vi "mod1 sub.vi"(3 "Modulname":string, 4 "Daten":string, 5 "Format":string="%d") -> (0 "Sperre":bool, 1 "Ausgang":string)   [LabVIEW 2010]
panel:
  out "Zykluslänge b":dbl
  out "Achtung":string
  out "Zykluslänge a":dbl
  out "Pre1A":dbl[][](array[numeric])
  out "TrapA":dbl[][](array[numeric]) format="%.2f"
  out "Main1A":dbl[][](array[numeric]) format="%.2f"
  out "MFC1":dbl[][](array[numeric]) format="%.2f"
  out "FanMain1":dbl[][](array[numeric])
  out "V1B":dbl[][](array[numeric]) format="%.2f"
  out "V1A":dbl[][](array[numeric])
  out "S1A1":dbl[][](array[numeric]) format="%.2f"
  out "pc1 C":dbl[][](array[numeric])
  out "pc1 A":dbl[][](array[numeric])
  in  "TrapA":bool
  in  "FanMain1A":bool
  in  "V1A":bool
  in  "V1B":bool
  in  "Main1A":bool
  in  "Pre1A":bool
  in  "MFC1":bool
  in  "S1A1":bool
  in  "pc1C":bool
  in  "pc1A":bool
  in  "Zurück":bool
  out "new picture":picture
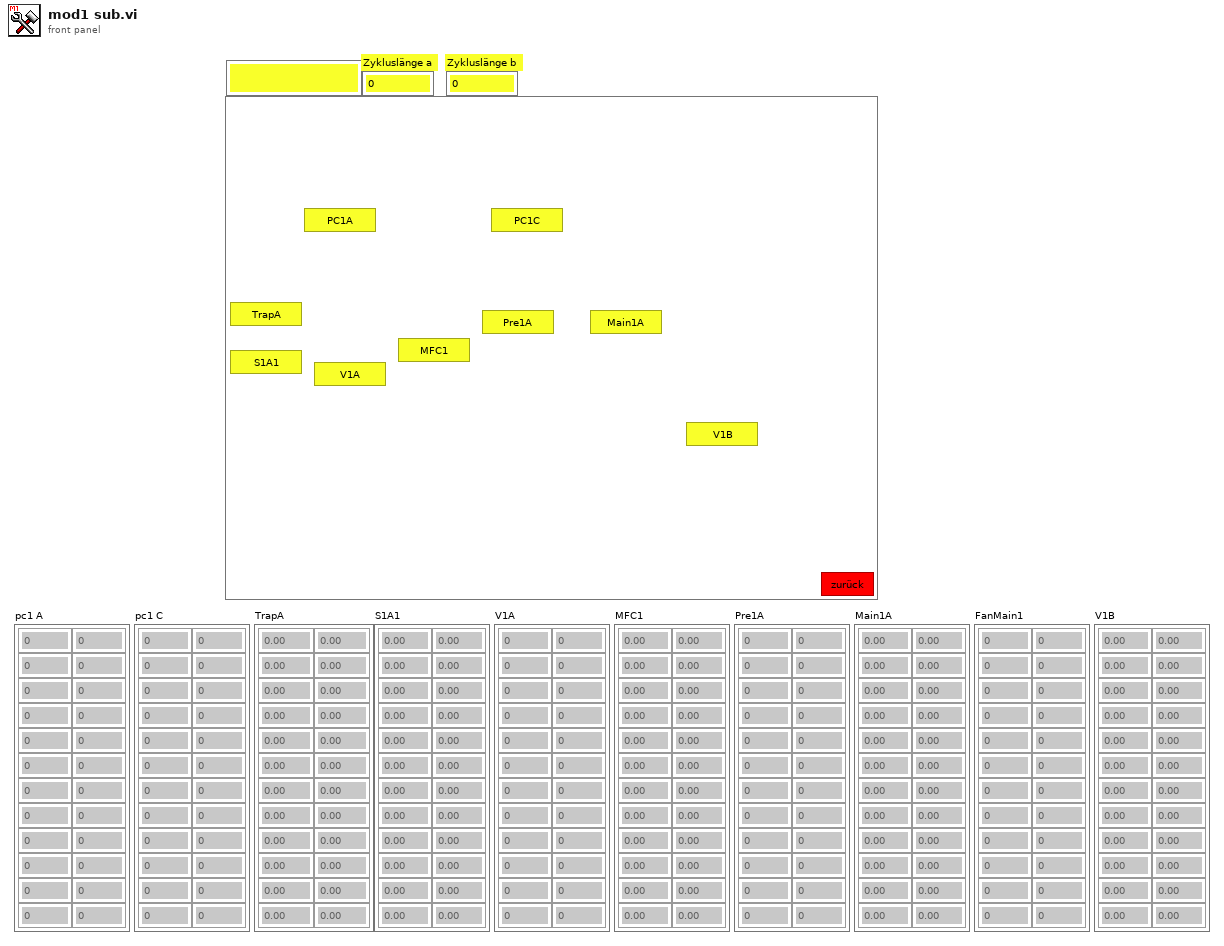
[diagram p1: front panel]
types:
  T1 = typedef "imagedata.ctl" = cluster{"image type":i32, "image depth":i32, "image":u8[], "mask":u8[], "colors":u32[], "Rectangle":cluster{"left":i16, "top":i16, "right":i16, "bottom":i16}}
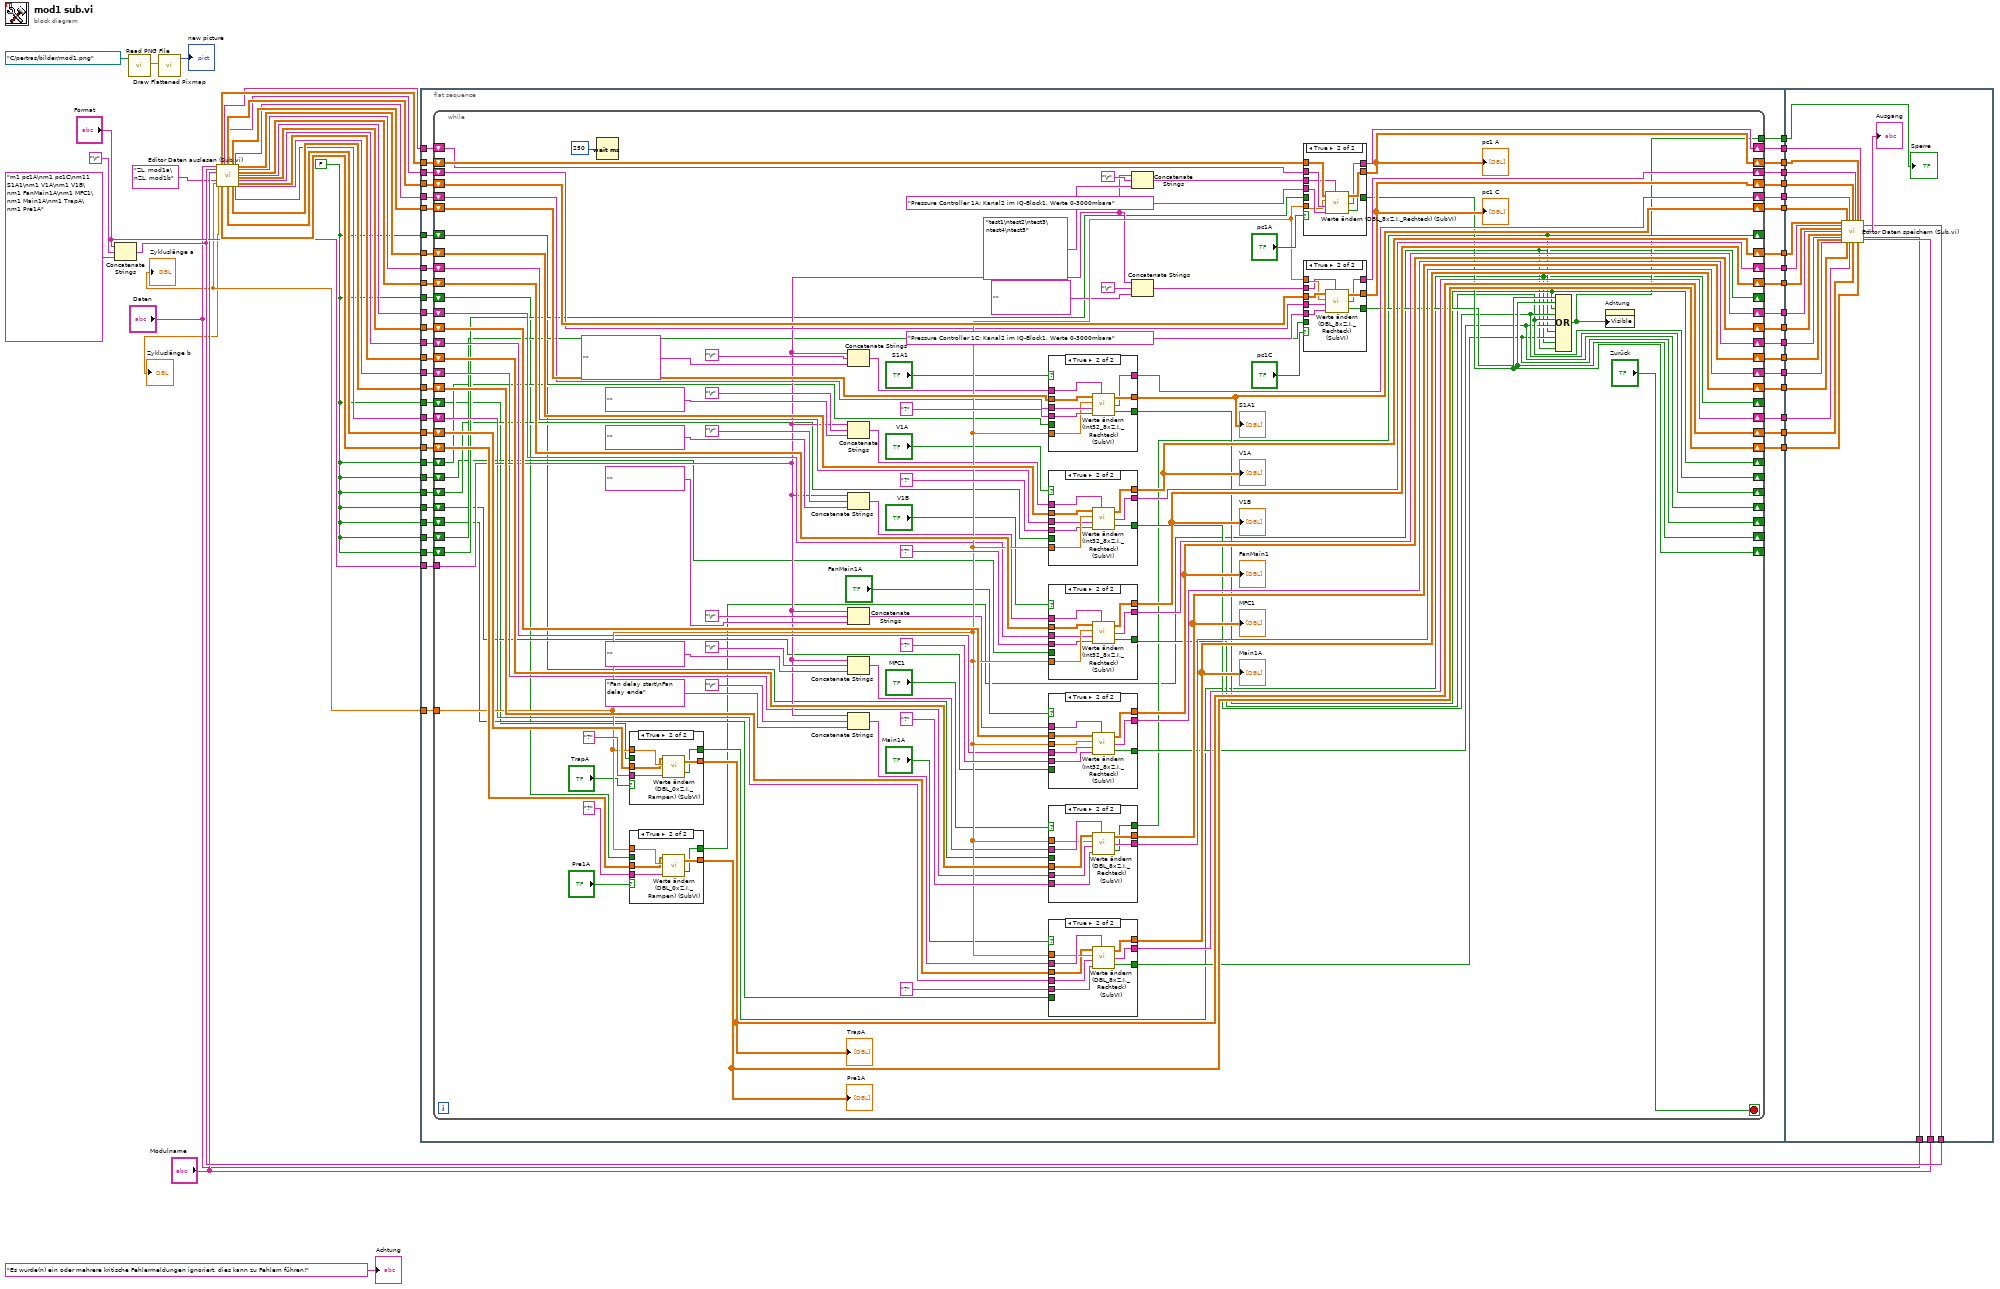
[diagram p0: block diagram]
diagram:
  w2 = FALSE
  n1 = Concatenate Strings("Format", "\r", "m1 pc1A\nm1 pc1C\nm11 S1A1\nm1 V1A\nm1 V1B\nm1 FanMain1A\nm1 MFC1\nm1 Main1A\nm1 TrapA\nm1 Pre1A" ("String")) -> (w38:string)
  n2 = call <vilib>:"Read PNG File.vi"("path to PNG file"=path "C:/pertras/bilder/mod1.png") -> ("image data"=w49:T1)  [unwired: 8 in, 2 out]
  n3 = call <vilib>:"Draw Flattened Pixmap.vi"("image data"=w49) -> ("new picture"=→"new picture":picture)  [unwired: 8 in]
  n4 = call "Editor Daten auslesen (Sub.vi).vi"("Daten"="Daten", "Formatierung+Namen"=w38, "Modulname"="Modulname", "Zykluslängen Namen"="ZL. mod1a\nZL. mod1b" ("Zykluslänge Name")) -> ("Zykluslänge 1"=w10:dbl, "Zykluslänge 2"=→"Zykluslänge b":dbl, "1"=w35:dbl[][], "10"=w21:dbl[][], "Z 1"=w34:string, "2"=w33:dbl[][], "9"=w22:dbl[][], "Z 2"=w32:string, "3"=w31:dbl[][], "8"=w23:dbl[][], "Z 3"=w30:string, "Z 8"=w5:string, "4"=w29:dbl[][], "Z 4"=w20:string, "5"=w28:dbl[][], "Z5"=w27:string, "6"=w26:dbl[][], "Z 6"=w25:string, "7"=w24:dbl[][], "Z 7"=w6:string)  [unwired: 2 in, 2 out]
  "Zykluslänge a" <- w10
  n5 = flat-sequence {
    tunnel: w10 -> [w100]
    tunnel: [w99] -> w48
    tunnel: [w98] -> w47
    tunnel: [w97] -> w46
    tunnel: [w96] -> w45
    tunnel: [w95] -> w44
    tunnel: [w94] -> w43
    tunnel: [w93] -> w42
    tunnel: [w92] -> w41
    tunnel: [w91] -> w40
    tunnel: [w90] -> w39
    tunnel: w35 -> [w89]
    tunnel: w34 -> [w88]
    tunnel: w33 -> [w87]
    tunnel: w32 -> [w86]
    tunnel: w31 -> [w85]
    tunnel: w30 -> [w84]
    tunnel: w29 -> [w83]
    tunnel: w28 -> [w82]
    tunnel: w27 -> [w81]
    tunnel: w26 -> [w80]
    tunnel: w25 -> [w79]
    tunnel: w24 -> [w78]
    tunnel: w23 -> [w77]
    tunnel: w22 -> [w76]
    tunnel: w21 -> [w75]
    tunnel: w20 -> [w74]
    tunnel: [w73] -> w19
    tunnel: [w72] -> w18
    tunnel: [w71] -> w17
    tunnel: [w70] -> w16
    tunnel: [w69] -> w15
    tunnel: [w68] -> w14
    tunnel: "Format" -> [w67]
    tunnel: [w66] -> w8
    tunnel: [w65] -> w7
    tunnel: w6 -> [w64]
    tunnel: w5 -> [w63]
    tunnel: [w62] -> w4
    tunnel: w2 -> [w61]
    tunnel: w2 -> [w60]
    tunnel: w2 -> [w59]
    tunnel: w2 -> [w58]
    tunnel: w2 -> [w57]
    tunnel: w2 -> [w56]
    tunnel: w2 -> [w55]
    tunnel: w2 -> [w54]
    tunnel: w2 -> [w53]
    tunnel: w2 -> [w52]
    tunnel: w48 -> [w328]
    tunnel: w47 -> [w322]
    tunnel: w46 -> [w327]
    tunnel: w45 -> [w319]
    tunnel: w44 -> [w326]
    tunnel: w43 -> [w316]
    tunnel: w42 -> [w325]
    tunnel: w41 -> [w314]
    tunnel: w40 -> [w313]
    tunnel: w39 -> [w324]
    tunnel: w38 -> [w329]
    tunnel: w19 -> [w323]
    tunnel: w18 -> [w321]
    tunnel: w17 -> [w320]
    tunnel: w16 -> [w318]
    tunnel: w15 -> [w317]
    tunnel: w14 -> [w315]
    tunnel: "Modulname" -> [w312]
    tunnel: "Daten" -> [w311]
    tunnel: w8 -> [w310]
    tunnel: w7 -> [w309]
    tunnel: w4 -> [w308]
    frame #0 {
      n6 = while {
        shift-right: [w172] -> w99
        shift-left: w89 -> [w202]
        tunnel: w100 -> [w181]
        shift-right: [w158] -> w98
        shift-left: w87 -> [w199]
        shift-right: [w171] -> w97
        shift-left: w85 -> [w189]
        shift-right: [w157] -> w96
        shift-left: w83 -> [w188]
        shift-right: [w170] -> w95
        shift-left: w82 -> [w187]
        shift-right: [w154] -> w94
        shift-left: w80 -> [w186]
        shift-right: [w169] -> w93
        shift-left: w78 -> [w185]
        shift-right: [w152] -> w92
        shift-left: w77 -> [w184]
        shift-right: [w151] -> w91
        shift-left: w76 -> [w183]
        shift-right: [w168] -> w90
        shift-left: w75 -> [w182]
        shift-right: [w161] -> w73
        shift-left: w88 -> [w167]
        shift-right: [w160] -> w72
        shift-left: w86 -> [w166]
        shift-right: [w159] -> w71
        shift-left: w84 -> [w165]
        shift-right: [w156] -> w70
        shift-left: w74 -> [w162]
        shift-right: [w155] -> w69
        shift-left: w81 -> [w164]
        shift-right: [w153] -> w68
        shift-left: w79 -> [w163]
        tunnel: w67 -> [w128]
        shift-right: [w125] -> w66
        shift-left: w64 -> [w124]
        shift-right: [w123] -> w65
        shift-left: w63 -> [w122]
        tunnel: [w103] -> w62
        shift-right: [w111] -> _
        shift-left: w61 -> [w121]
        shift-right: [w110] -> _
        shift-left: w60 -> [w120]
        shift-right: [w109] -> _
        shift-left: w59 -> [w119]
        shift-right: [w108] -> _
        shift-left: w58 -> [w118]
        shift-right: [w107] -> _
        shift-left: w57 -> [w117]
        shift-right: [w106] -> _
        shift-left: w56 -> [w116]
        shift-right: [w105] -> _
        shift-left: w55 -> [w115]
        shift-right: [w104] -> _
        shift-left: w54 -> [w114]
        shift-right: [w101] -> _
        shift-left: w53 -> [w112]
        shift-right: [w102] -> _
        shift-left: w52 -> [w113]
        stop <- "Zurück" stop-if-true
        n7 = Wait (ms)(milliseconds to wait=u32 250 ("Zu wartende ms")) -> ()  [unwired: 1 out]
        n8 = case shown="True" "TrapA" {
          tunnel: "?" -> [_ w216]
          tunnel: w183 -> [w214 w217]
          tunnel: w181 -> [_ w218]
          tunnel: [w214 w219] -> w151
          tunnel: [w213 w215] -> w102
          tunnel: w113 -> [w213 _]
          frame False {
          }
          frame True {
            n9 = call "Werte ändern (DBL_0xZ.I._Rampen) (SubVI).vi"("geladene Werte (Zeit (s); Wert)"=w217, "Zykluslänge"=w218, "Info"=w216) -> ("Ausgang"=w219:dbl[][], "Sperre"=w215:bool)  [unwired: 2 in]
          }
        }
        "TrapA" <- w151
        n10 = case shown="True" "Pre1A" {
          tunnel: [w207 w209] -> w168
          tunnel: "?" -> [_ w210]
          tunnel: w182 -> [w207 w211]
          tunnel: w181 -> [_ w212]
          tunnel: w112 -> [w206 _]
          tunnel: [w206 w208] -> w101
          frame False {
          }
          frame True {
            n11 = call "Werte ändern (DBL_0xZ.I._Rampen) (SubVI).vi"("geladene Werte (Zeit (s); Wert)"=w211, "Zykluslänge"=w212, "Info"=w210) -> ("Ausgang"=w209:dbl[][], "Sperre"=w208:bool)  [unwired: 2 in]
          }
        }
        "Pre1A" <- w168
        n12 = Concatenate Strings(w128, "\r", "") -> (w136:string)
        n13 = Concatenate Strings(w128, "\r", "") -> (w135:string)
        n14 = Concatenate Strings(w128, "\r", "") -> (w134:string)
        n15 = Concatenate Strings(w128, "\r", "") -> (w133:string)
        n16 = Concatenate Strings(w128, "\r", "") -> (w127:string)
        n17 = Concatenate Strings(w128, "\r", "Fan delay start\nFan delay ende") -> (w126:string)
        n18 = case shown="True" "S1A1" {
          tunnel: [w277 w285] -> w171
          tunnel: "?" -> [_ w283]
          tunnel: w189 -> [w277 w280]
          tunnel: w181 -> [_ w281]
          tunnel: w165 -> [w276 w282]
          tunnel: [w276 w284] -> w159
          tunnel: w136 -> [_ w279]
          tunnel: [w275 w278] -> w109
          tunnel: w119 -> [w275 _]
          frame False {
          }
          frame True {
            n19 = call "Werte ändern (Int32_8xZ.I._Rechteck) (SubVI).vi"("geladene Werte (Zeit (s); Wert)"=w280, "Zykluslänge"=w281, "Z.I."=w282, "Info"=w283, "Format+Namen"=w279) -> ("Ausgang"=w285:dbl[][], "Z.I."=w284:string, "Sperre"=w278:bool)
          }
        }
        "S1A1" <- w171
        n20 = case shown="True" "V1A" {
          tunnel: "?" -> [_ w271]
          tunnel: w188 -> [w266 w273]
          tunnel: w181 -> [_ w274]
          tunnel: w162 -> [w265 w272]
          tunnel: [w266 w269] -> w157
          tunnel: [w265 w270] -> w156
          tunnel: w135 -> [_ w268]
          tunnel: [w264 w267] -> w108
          tunnel: w118 -> [w264 _]
          frame False {
          }
          frame True {
            n21 = call "Werte ändern (Int32_8xZ.I._Rechteck) (SubVI).vi"("geladene Werte (Zeit (s); Wert)"=w273, "Zykluslänge"=w274, "Z.I."=w272, "Info"=w271, "Format+Namen"=w268) -> ("Ausgang"=w269:dbl[][], "Z.I."=w270:string, "Sperre"=w267:bool)
          }
        }
        "V1A" <- w157
        n22 = case shown="True" "V1B" {
          tunnel: [w255 w263] -> w170
          tunnel: "?" -> [_ w258]
          tunnel: w187 -> [w255 w260]
          tunnel: w181 -> [_ w261]
          tunnel: w164 -> [w254 w259]
          tunnel: [w254 w262] -> w155
          tunnel: w134 -> [_ w257]
          tunnel: [w253 w256] -> w107
          tunnel: w117 -> [w253 _]
          frame False {
          }
          frame True {
            n23 = call "Werte ändern (Int32_8xZ.I._Rechteck) (SubVI).vi"("geladene Werte (Zeit (s); Wert)"=w260, "Zykluslänge"=w261, "Z.I."=w259, "Info"=w258, "Format+Namen"=w257) -> ("Ausgang"=w263:dbl[][], "Z.I."=w262:string, "Sperre"=w256:bool)
          }
        }
        "V1B" <- w170
        n24 = case shown="True" "FanMain1A" {
          tunnel: "?" -> [_ w251]
          tunnel: w186 -> [w244 w249]
          tunnel: w181 -> [_ w250]
          tunnel: w163 -> [w243 w252]
          tunnel: [w244 w248] -> w154
          tunnel: [w243 w247] -> w153
          tunnel: w133 -> [_ w246]
          tunnel: [w242 w245] -> w106
          tunnel: w116 -> [w242 _]
          frame False {
          }
          frame True {
            n25 = call "Werte ändern (Int32_8xZ.I._Rechteck) (SubVI).vi"("geladene Werte (Zeit (s); Wert)"=w249, "Zykluslänge"=w250, "Z.I."=w252, "Info"=w251, "Format+Namen"=w246) -> ("Ausgang"=w248:dbl[][], "Z.I."=w247:string, "Sperre"=w245:bool)
          }
        }
        "FanMain1" <- w154
        n26 = case shown="True" "MFC1" {
          tunnel: [w233 w240] -> w169
          tunnel: "?" -> [_ w237]
          tunnel: w185 -> [w233 w239]
          tunnel: w181 -> [_ w238]
          tunnel: w127 -> [_ w241]
          tunnel: [w232 w236] -> w125
          tunnel: w124 -> [w232 w235]
          tunnel: [w231 w234] -> w105
          tunnel: w115 -> [w231 _]
          frame False {
          }
          frame True {
            n27 = call "Werte ändern (DBL_8xZ.I._Rechteck) (SubVI).vi"("geladene Werte (Zeit (s); Wert)"=w239, "Zykluslänge"=w238, "Z.I."=w235, "Info"=w237, "Format+Namen"=w241) -> ("Ausgang"=w240:dbl[][], "Z.I."=w236:string, "Sperre"=w234:bool)
          }
        }
        "MFC1" <- w169
        n28 = case shown="True" "Main1A" {
          tunnel: "?" -> [_ w228]
          tunnel: w184 -> [w222 w226]
          tunnel: w181 -> [_ w227]
          tunnel: [w222 w229] -> w152
          tunnel: w126 -> [_ w230]
          tunnel: [w221 w225] -> w123
          tunnel: w122 -> [w221 w224]
          tunnel: [w220 w223] -> w104
          tunnel: w114 -> [w220 _]
          frame False {
          }
          frame True {
            n29 = call "Werte ändern (DBL_8xZ.I._Rechteck) (SubVI).vi"("geladene Werte (Zeit (s); Wert)"=w226, "Zykluslänge"=w227, "Z.I."=w224, "Info"=w228, "Format+Namen"=w230) -> ("Ausgang"=w229:dbl[][], "Z.I."=w225:string, "Sperre"=w223:bool)
          }
        }
        "Main1A" <- w152
        n30 = Concatenate Strings(w128, "\r", "test1\ntest2\ntest3\ntest4\ntest5") -> (w150:string)
        n31 = Concatenate Strings(w128, "\r", "") -> (w137:string)
        n32 = case shown="True" "pc1A" {
          tunnel: w202 -> [w299 w305]
          tunnel: [w299 w302] -> w172
          tunnel: w181 -> [_ w304]
          tunnel: "Pressure Controller 1A: Kanal2 im IQ-Block1, Werte 0-3000mbara" -> [_ w307]
          tunnel: w167 -> [w298 w306]
          tunnel: [w298 w301] -> w161
          tunnel: w150 -> [_ w303]
          tunnel: [w297 w300] -> w111
          tunnel: w121 -> [w297 _]
          frame False {
          }
          frame True {
            n33 = call "Werte ändern (DBL_8xZ.I._Rechteck) (SubVI).vi"("geladene Werte (Zeit (s); Wert)"=w305, "Zykluslänge"=w304, "Z.I."=w306, "Info"=w307, "Format+Namen"=w303) -> ("Ausgang"=w302:dbl[][], "Z.I."=w301:string, "Sperre"=w300:bool)
          }
        }
        "pc1 A" <- w172
        n34 = case shown="True" "pc1C" {
          tunnel: "Pressure Controller 1C: Kanal2 im IQ-Block1, Werte 0-3000mbara" -> [_ w290]
          tunnel: w181 -> [_ w293]
          tunnel: w199 -> [w288 w294]
          tunnel: w166 -> [w287 w292]
          tunnel: [w288 w296] -> w158
          tunnel: [w287 w295] -> w160
          tunnel: w137 -> [_ w291]
          tunnel: [w286 w289] -> w110
          tunnel: w120 -> [w286 _]
          frame False {
          }
          frame True {
            n35 = call "Werte ändern (DBL_8xZ.I._Rechteck) (SubVI).vi"("geladene Werte (Zeit (s); Wert)"=w294, "Zykluslänge"=w293, "Z.I."=w292, "Info"=w290, "Format+Namen"=w291) -> ("Ausgang"=w296:dbl[][], "Z.I."=w295:string, "Sperre"=w289:bool)
          }
        }
        "pc1 C" <- w158
        n36 = Compound Arithmetic op=OR(w111, w110, w109, w108, w107, w106, w105, w104, w102, w101) -> (w103:bool)
        n37 = property on="Achtung" class="Str"("Visible"=w103) -> ()  [unwired: 2 in, 2 out]
      }
    }
    frame #1 {
      n38 = call "Editor Daten speichern (Sub.vi).vi"("4"=w319, "Z 4"=w318, "5"=w326, "Z 5"=w317, "6"=w316, "Z 6"=w315, "7"=w325, "Z 7"=w310, "3"=w327, "8"=w314, "Z 3"=w320, "Z 8"=w309, "2"=w322, "9"=w313, "Z 2"=w321, "1"=w328, "10"=w324, "Z 1"=w323, "Formatierung+Namen"=w329, "Daten"=w311, "Modulname"=w312) -> ("Ausgang"=→"Ausgang":string)  [unwired: 6 in]
      "Sperre" <- w308
    }
  }
  "Achtung" <- "Es wurde(n) ein oder mehrere kritische Fehlermeldungen ignoriert, dies kann zu Fehlern führen!"
